vi "Create List.vi"(7 "List Implementation (Array)":refnum<class "ListImp.lvclass">, 8 "error in (no error)":errorcluster) -> (0 "error out":errorcluster, 3 "List out":refnum<class "List.lvclass">)   [LabVIEW 2017, in "LapDog.Collections.v0.Lists.lvlib" / "List.lvclass"]
doc: "Creates a List object. Wire a List Implementation object cube to the List Implementation input terminal to use an implementation other than the default array implementation. This method will automatically invoke the Create method for the implementation object.\n\nThis method returns a default List object if an error is on the input terminal."
uses:
  List.lvclass
  ListImp/ListImp.lvclass
  List.lvclass/List.ctl
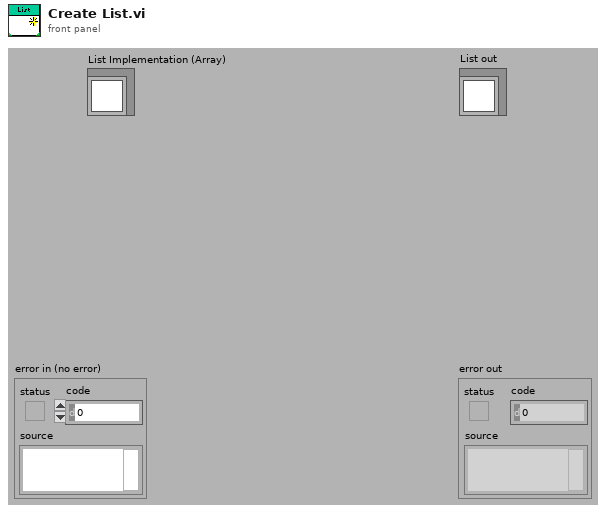
[diagram p1: front panel]
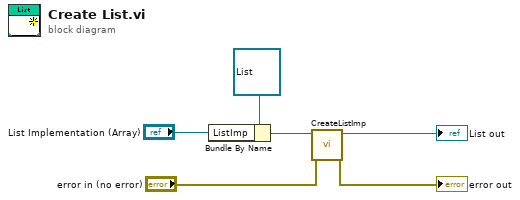
[diagram p0: block diagram]
diagram:
  n1 = Bundle By Name(cluster=refnum<class "List.lvclass"> refnum ("List in"), "ListImp"="List Implementation (Array)") -> (w4:refnum<class "List.lvclass">)
  n2 = call "CreateListImp.vi"("error in (no error)"="error in (no error)", "List in"=w4) -> ("error out"=→"error out":errorcluster, "List out"=→"List out":refnum<class "List.lvclass">)  [unwired: 8 in]
